vi "Pnumatics gear actuator-firstVI.vi"() -> ()   [LabVIEW 2016]
uses:
  <vilib>/Rock Robotics/WPI/Solenoid/WPI_SolenoidDevRef.ctl
  <vilib>/Rock Robotics/WPI/Solenoid/WPI_SolenoidChannel.ctl
  <userlib>/836-Libraries/Pneumatics/Support_Code/Solenoid_Configure.ctl
  <userlib>/836-Libraries/Pneumatics/Support_Code/Pneumatics_Configuration.ctl
  <userlib>/836-Libraries/Pneumatics/Support_Code/Feedback_Method.ctl
panel:
  in  "SolenoidDevRef 2":T1
  in  "SolenoidDevRef":T1
  in  "name (unnamed) 2":string
  in  "name (unnamed)":string
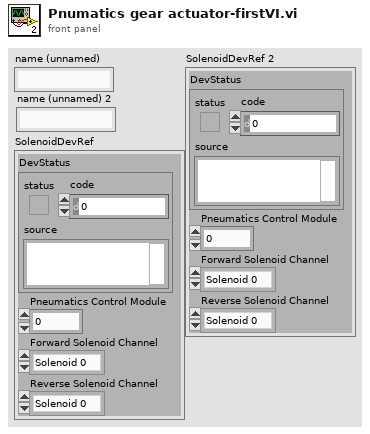
[diagram p1: front panel]
types:
  T1 = typedef "WPI_SolenoidDevRef.ctl" = cluster{"DevStatus":errorcluster, "Pneumatics Control Module":u8, "Forward Solenoid Channel":T2, "Reverse Solenoid Channel":T2}
  T2 = typedef "WPI_SolenoidChannel.ctl" = enum8{"Solenoid 0", "Solenoid 1", "Solenoid 2", "Solenoid 3", "Solenoid 4", "Solenoid 5", "Solenoid 6", "Solenoid 7", "Invalid"}
  T3 = typedef "Solenoid_Configure.ctl" = cluster{"Normal Timing":T4, "Feedback Forward":T5, "Feedback Reverse":T5, "Analog Thresholds":T4, "Timeout":T4}
  T4 = typedef "Pneumatics_Configuration.ctl" = cluster{"Forward":dbl, "Reverse":dbl}
  T5 = typedef "Feedback_Method.ctl" = enum16{"Timed", "Analog", "Digital", "Analog (Inverted)", "Digital (Inverted)"}
  T6 = typedef "Pneumatic_Sensor_Loop.ctl" = cluster{"Status Queue":refnum<queue>, "Status Loop":refnum<k33>, "Relay Value":T7}
  T7 = typedef "WPI_SolenoidValue.ctl" = enum16{"Off", "On", "Forward", "Reverse"}
  T8 = typedef "Solenoid_Control_Loop.ctl" = cluster{"Control Notifier":refnum<notifier>, "Initial Position":T9, "SolenoidDevRef":T1, "Status Loop":refnum<k33>}
  T9 = typedef "Pneumatics_Position.ctl" = enum16{"Forward", "Reverse"}
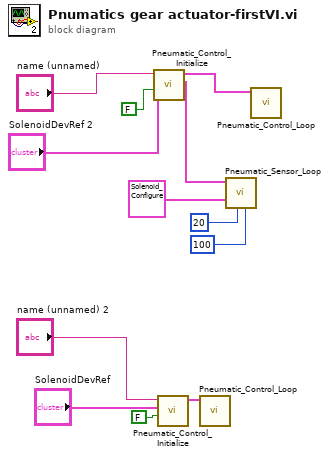
[diagram p0: block diagram]
diagram:
  n1 = call <userlib>:"Pneumatic_Control_Initialize.vi"("Forward?"=FALSE, "SolenoidDevRef"="SolenoidDevRef 2", "name (unnamed)"="name (unnamed)") -> ("Sense Loop"=w11:T6, "Control Loop"=w12:T8)  [unwired: 7 in]
  n2 = call <userlib>:"Pneumatic_Control_Initialize.vi"("Forward?"=FALSE, "SolenoidDevRef"="SolenoidDevRef", "name (unnamed)"="name (unnamed) 2") -> ("Control Loop"=w6:T8)  [unwired: 7 in, 1 out]
  n3 = call <userlib>:"Pneumatic_Control_Loop.vi"("Cluster in"=w6) -> ()  [unwired: 11 in]
  n4 = call <userlib>:"Pneumatic_Sensor_Loop.vi"("Priority"=100, "Period"=i64 20, "Solenoid Configuration"=T3 {"Normal Timing"={"Forward"=2000.0, "Reverse"=2000.0}, "Feedback Forward"=enum."Timed", "Feedback Reverse"=enum."Timed", "Analog Thresholds"={"Forward"=0.0, "Reverse"=0.0}, "Timeout"={"Forward"=0.0, "Reverse"=0.0}}, "Cluster"=w11) -> ()  [unwired: 8 in]
  n5 = call <userlib>:"Pneumatic_Control_Loop.vi"("Cluster in"=w12) -> ()  [unwired: 11 in]
